vi "Dialog Box Timeout v2.vi"(8 "Error In":errorcluster, 10 "Timeout (s)":dbl=5.0 caption="Time Target (s)", 11 "Message":string="Message") -> (0 "Error Out":errorcluster)   [LabVIEW 2019]
doc: "Developed by Kevin Thompson\nkevin@thompsonengineering.net\n\nCopyright 2018-2020\nThompson Engineering, LLC\nDisplays a dialog box that contains a message and a single \"OK\" button using the One Button Dialog VI. This VI will automatically press \"OK\" after Timeout (s) has occurred."
uses:
  user32.dll
panel:
  in  "Stopped":bool
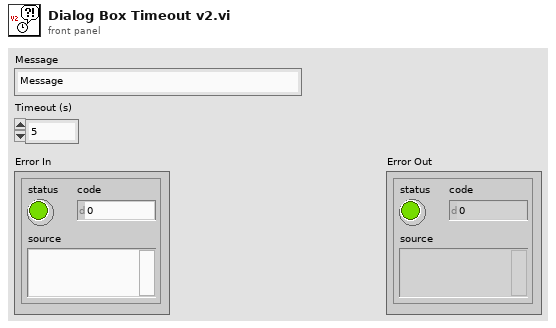
[diagram p1: front panel]
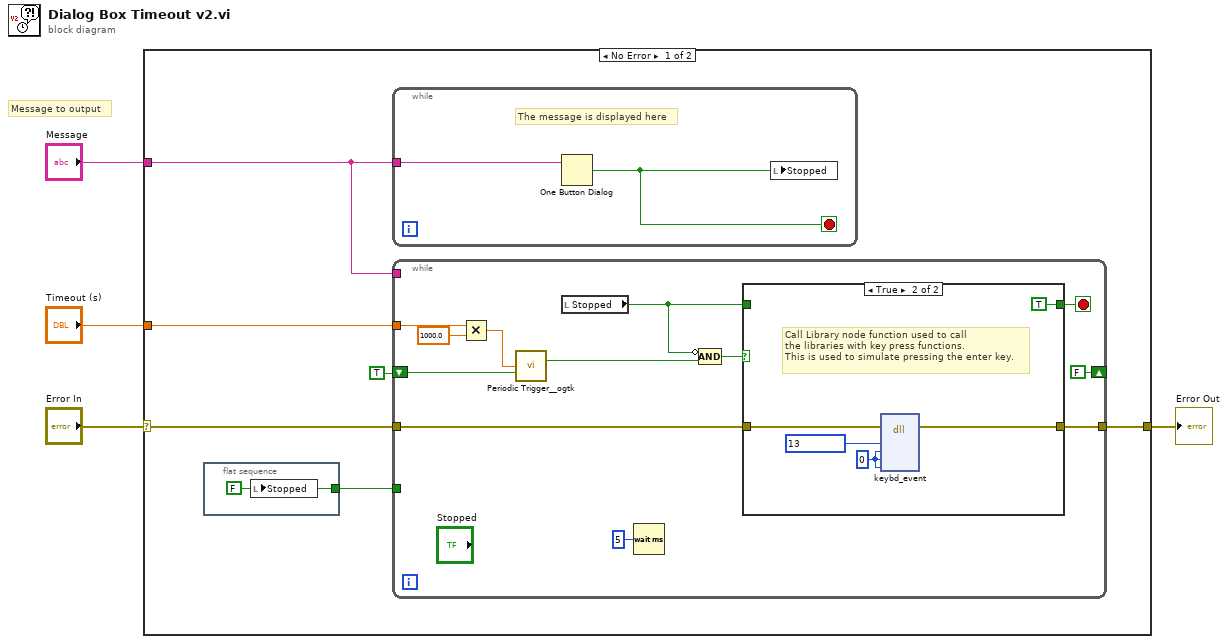
[diagram p0: block diagram]
diagram:
  # "Message to output"
  n1 = case shown="No Error" "Error In" {
    selector: "Error In" -> [w8 w33]
    tunnel: [w7 w33] -> w4
    tunnel: "Message" -> [w10 _]
    tunnel: "Timeout (s)" -> [w9 _]
    frame No Error {
      n2 = flat-sequence {
        tunnel: [w11] -> w5
        frame #0 {
          w11 = FALSE ("Stopped")
          n3 = local write "Stopped"(w11) -> ()
        }
      }
      n4 = while {
        tunnel: w10 -> [w32]
        stop <- w31 stop-if-true
        # "The message is displayed here"
        n5 = One Button Dialog(message=w32) -> (true=w31:bool)  [unwired: 1 in]
        n6 = local write "Stopped"(w31) -> ()
      }
      n7 = while {
        tunnel: w10 -> [_]
        tunnel: w9 -> [w17]
        tunnel: w8 -> [w13]
        tunnel: [w20] -> w7
        shift-right: [FALSE] -> _
        shift-left: TRUE -> [w16]
        tunnel: w5 -> [_]
        stop <- w21 stop-if-true
        n8 = Multiply(x=w17, y=1000.0) -> (x*y=w19:dbl)
        n9 = call <userlib>:"Periodic Trigger__ogtk.vi"("time (ms)"=w19, "reset"=w16) -> ("Triggered"=w15:bool)  [unwired: 11 in, 2 out]
        n10 = local read "Stopped"() -> (w12:bool)
        n11 = Wait (ms)(milliseconds to wait=u32 5) -> ()  [unwired: 1 out]
        n12 = Compound Arithmetic op=AND(invert w12, w15) -> (w23:bool)
        n13 = case shown="True" w23 {
          tunnel: [w25 TRUE] -> w21
          tunnel: w12 -> [w25 _]
          tunnel: w13 -> [w24 w27]
          tunnel: [w24 w26] -> w20
          frame False {
          }
          frame True {
            w29 = u8 0 ("b scan")
            # "Call Library node function used to call \nthe libraries with key press functions. \nThis is used to simulate pressing the enter key."
            n14 = dll-call lib="user32.dll" fn="keybd_event" label="user32.dll: keybd_event"(error in=w27, "bVk"=u8 13 ("Virtual Key"), "bScan"=w29, "dwFlags"=w29, "dwExtraInfo"=w29) -> (error out=w26:errorcluster)  [unwired: 7 in, 1 out]
          }
        }
      }
    }
    frame Error {
      # "If an error has occurred, do not run dialog box and return error to main VI"
    }
  }
  "Error Out" <- w4
